vi "PowerUp.vi"(1 "初始DO参数":string[][](array[string])=[["/port2/line0", ""], ["/port2/line3", "/port2/line6"], ["/port0/line31", ""]], 2 "索引Index":i32[](array[numeric]), 3 "NewVal":bool, 4 "DaqmxName":string) -> ()   [LabVIEW 2013]
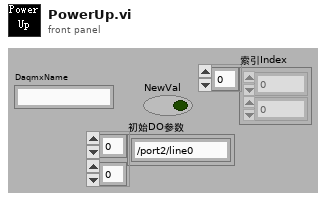
[diagram p1: front panel]
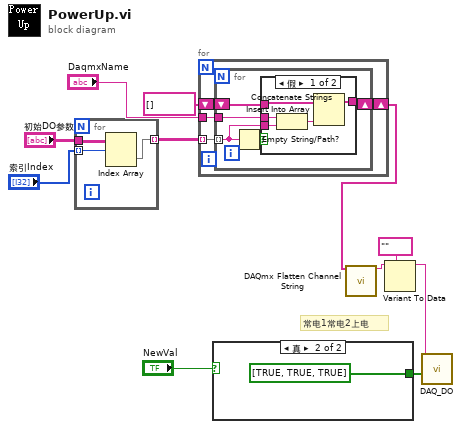
[diagram p0: block diagram]
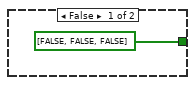
[diagram p3: hidden frame]
diagram:
  # "常电1常电2上电"
  n1 = for {
    tunnel: "初始DO参数" -> [w14]
    tunnel: [w13] -> w2 mode=indexing
    tunnel: "索引Index" -> [w12] mode=indexing
    n2 = Index Array(array=w14, index (row)=w12) -> (element=w13:string[])  [unwired: 1 in]
  }
  n3 = for {
    tunnel: "DaqmxName" -> [w18]
    tunnel: w2 -> [w15] mode=indexing
    shift-right: [w17] -> w5
    shift-left: string[] [] -> [w16]
    n4 = for {
      tunnel: w18 -> [w23]
      tunnel: w15 -> [w21] mode=indexing
      shift-right: [w19] -> w17
      shift-left: w16 -> [w20]
      n5 = Empty String/Path?(string/path=w21) -> (empty?=w22:bool)
      n6 = case shown="假" w22 {
        tunnel: w23 -> [w28 _]
        tunnel: w21 -> [w27 _]
        tunnel: w20 -> [w25 w29]
        tunnel: [w24 w29] -> w19
        frame False {
          n7 = Concatenate Strings(w28, w27) -> (w26:string)
          n8 = Insert Into Array(array=w25, new element=w26) -> (w24:string[])  [unwired: 1 in]
        }
        frame True {
        }
      }
    }
  }
  n9 = case shown="真" "NewVal" {
    tunnel: [bool[] [FALSE, FALSE, FALSE] ("Bool") bool[] [TRUE, TRUE, TRUE] ("Bool")] -> w8
    frame False {
    }
    frame True {
    }
  }
  n10 = call <vilib>:"DAQmx Flatten Channel String.vi"("names in"=w5) -> ("names out"=w9:string)  [unwired: 13 in, 1 out]
  n11 = Variant To Data(type=tag "" ("lines"), Variant=w9) -> (data=w11:tag)  [unwired: 1 in, 1 out]
  n12 = call "DAQ_DO.vi"("Bool"=w8, "lines"=w11) -> ()  [unwired: 8 in, 2 out]
